vi "Add FPGA Hardware_Add FPGA.vi"(8 "error in (no error)":errorcluster, 9 "FPGA Settings":T1={"Path"=path "", "RIO Name"="RIO0", "Aliases"=[]}, 11 "FPGA Ref":refnum<k24>) -> (0 "error out":errorcluster, 3 "FPGA Ref out":refnum<k24>)   [LabVIEW 2019, in "Simple SysDef API.lvlib"]
uses:
  <userlib>/SimpleSysDef/Simple SysDef API.lvlib
  NationalInstruments.VeriStand.SystemDefinitionAPI
  <userlib>/SimpleSysDef/_SubVIs/Add FPGA Hardware_Settings.ctl
panel:
  # "5F92BE66-C305-11DD-B8A3-E45255D89593"
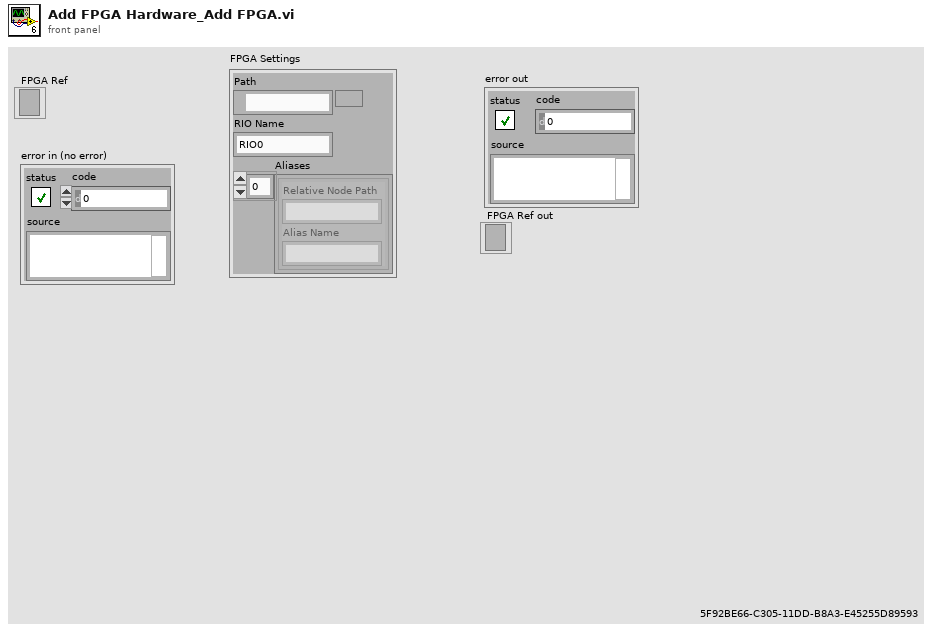
[diagram p1: front panel]
types:
  T1 = typedef "Simple SysDef API.lvlib/Add FPGA Hardware_Settings.ctl" = cluster{"Path":path, "RIO Name":string, "Aliases":cluster{"Relative Node Path":string, "Alias Name":string}[]}
  T2 = cluster{"Relative Node Path":string, "Alias Name":string}[]
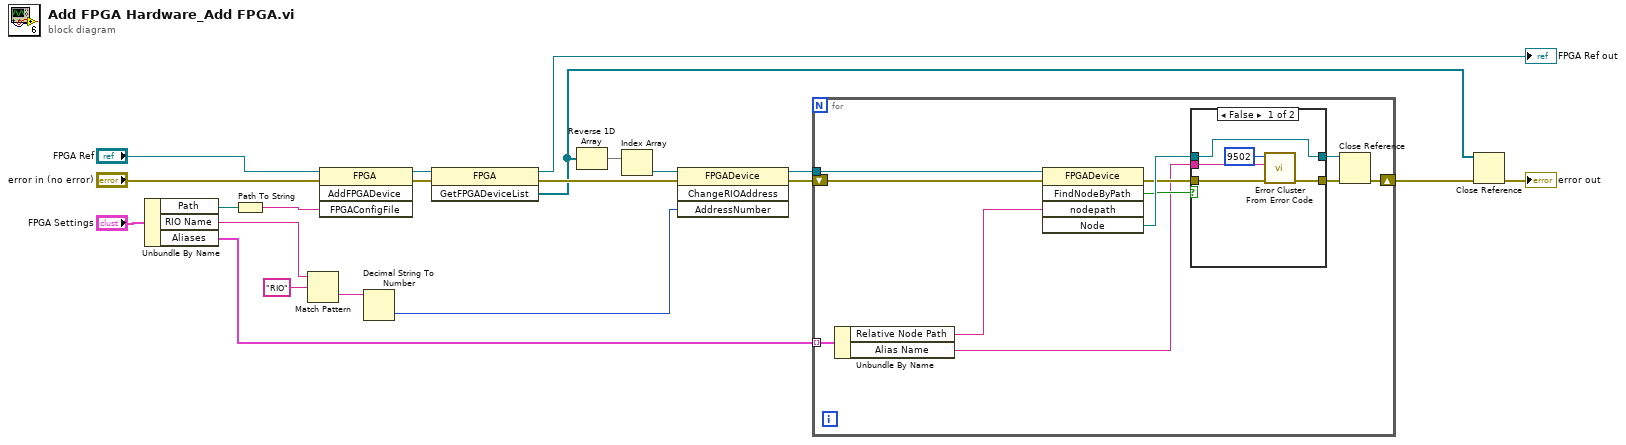
[diagram p0: block diagram]
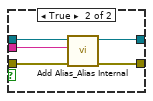
[diagram p2: hidden frame]
diagram:
  n1 = Unbundle By Name("FPGA Settings") -> ("Path"=w11:path, "RIO Name"=w10:string, "Aliases"=w7:T2)
  n2 = Path To String(path=w11) -> (string=w21:string)
  n3 = Match Pattern(string=w10, regular expression="RIO") -> (after substring=w16:string)  [unwired: 1 in, 3 out]
  n4 = invoke class="FPGA" method="AddFPGADevice"(reference="FPGA Ref", error in="error in (no error)", "FPGAConfigFile"=w21) -> (reference out=w19:refnum<k24>, error out=w20:errorcluster)  [unwired: 1 in, 2 out]
  n5 = Decimal String To Number(string=w16) -> (number=w15:i32)  [unwired: 2 in, 1 out]
  n6 = invoke class="FPGA" method="GetFPGADeviceList"(reference=w19, error in=w20) -> (reference out=→"FPGA Ref out":refnum<k24>, error out=w14:errorcluster, "GetFPGADeviceList"=w4:refnum<k24>[])  [unwired: 1 in]
  n7 = Reverse 1D Array(array=w4) -> (reversed array=w2:refnum<k24>[])
  n8 = Index Array(array=w2) -> (element=w3:refnum<k24>)  [unwired: 1 in]
  n9 = invoke class="FPGADevice" method="ChangeRIOAddress"(reference=w3, error in=w14, "AddressNumber"=w15) -> (reference out=w9:refnum<k24>, error out=w8:errorcluster)  [unwired: 1 in, 2 out]
  n10 = for {
    tunnel: w9 -> [w22]
    shift-right: [w28] -> w1
    shift-left: w8 -> [w23]
    tunnel: w7 -> [w27] mode=indexing
    n11 = Unbundle By Name(w27) -> ("Relative Node Path"=w24:string, "Alias Name"=w25:string)
    n12 = invoke class="FPGADevice" method="FindNodeByPath"(reference=w22, error in=w23, "nodepath"=w24) -> (error out=w31:errorcluster, "FindNodeByPath"=w26:bool, "Node"=w32:refnum<k24>)  [unwired: 2 in, 2 out]
    n13 = case shown="False" w26 {
      tunnel: w32 -> [w33 w42]
      tunnel: w31 -> [w36 w41]
      tunnel: [w33 w40] -> w30
      tunnel: [w35 w39] -> w29
      tunnel: w25 -> [w34 w38]
      frame False {
        n14 = call <userlib>:"Error Cluster From Error Code.vi"("error in (no error)"=w36, "error message (\"\")"=w34, "error code (0)"=9502) -> ("error out"=w35:errorcluster)  [unwired: 6 in]
      }
      frame True {
        n15 = call <userlib>:"Add Alias_Alias Internal.vi"("error in (no error)"=w41, "Name"=w38, "Base Node"=w42) -> ("error out"=w39:errorcluster, "Base Node out"=w40:refnum<k24>)  [unwired: 7 in]
      }
    }
    n16 = Close Reference(reference=w30, error in (no error)=w29) -> (error out=w28:errorcluster)
  }
  n17 = Close Reference(reference=w4, error in (no error)=w1) -> (error out=→"error out":errorcluster)
